vi "DevB.Read Message.vi"(8 "error in (no error)":errorcluster, 10 "timeout in ms (-1)":i32=-1, 11 "DevB Session in":T2) -> (0 "error out":errorcluster, 1 "type":T1, 2 "data":variant, 3 "DevB Session out":T2)   [LabVIEW 2018]
uses:
  typedefs/DevB.Message Session.ctl
  typedefs/DevB.Message.ctl
  typedefs/DevB.Message type.ctl
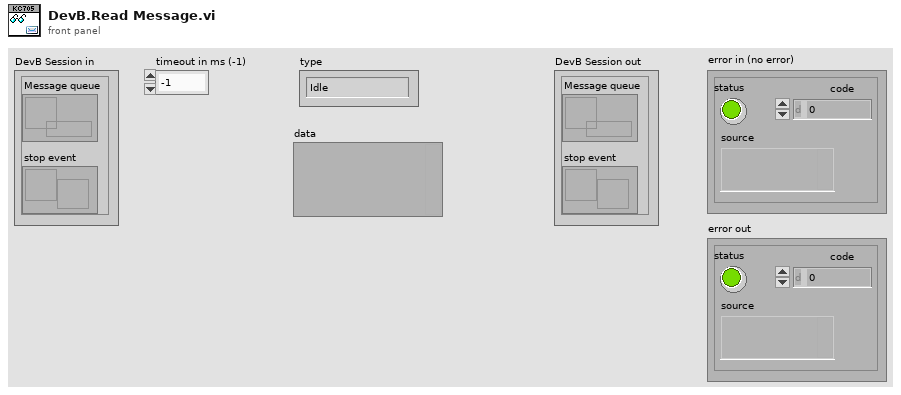
[diagram p1: front panel]
types:
  T1 = typedef "DevB.Message type.ctl" = enum16{"Idle", "Set Duration", "Set Frequency", "Set Phase", "Set Delay", "on/off", "check status"}
  T2 = typedef "DevB.Message Session.ctl" = cluster{"Message queue":refnum<queue>, "stop event":refnum<user-event>}
  T3 = typedef "DevB.Message.ctl" = cluster{"type":T1, "data":variant}
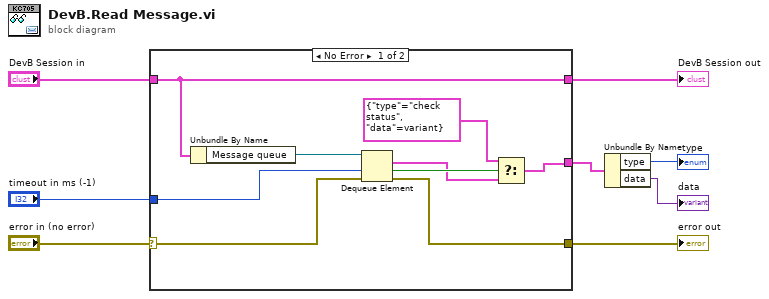
[diagram p0: block diagram]
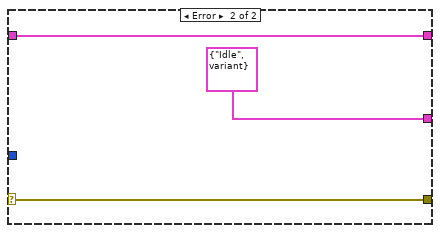
[diagram p2: hidden frame]
diagram:
  n1 = case shown="No Error" "error in (no error)" {
    selector: "error in (no error)" -> [w15 w20]
    tunnel: "DevB Session in" -> [w17 w19]
    tunnel: [w17 w19] -> w6
    tunnel: [w14 w20] -> w5
    tunnel: "timeout in ms (-1)" -> [w13 _]
    tunnel: [w10 T3 {"type"=enum."Idle", "data"=variant} ("DevB.Message")] -> w3
    frame No Error {
      n2 = Unbundle By Name(w17) -> ("Message queue"=w16:refnum<queue>)
      n3 = Dequeue Element(queue=w16, timeout in ms (-1)=w13, error in (no error)=w15) -> (element=w11:T3, timed out?=w12:bool, error out=w14:errorcluster)  [unwired: 1 out]
      n4 = Select(t=T3 {"type"=enum."check status", "data"=variant}, s=w12, f=w11) -> (s? t:f=w10:T3)
    }
    frame Error {
    }
  }
  "DevB Session out" <- w6
  "error out" <- w5
  n5 = Unbundle By Name(w3) -> ("type"=→"type":T1, "data"=→"data":variant)
